vi "lib TID Path.vi"(8 "error in (no error)":errorcluster, 10 "tid":string, 11 "data path":path) -> (0 "error out":errorcluster, 1 "description":string, 2 "date":string, 3 "tid path":path, 4 "size":i64)   [LabVIEW 2014]
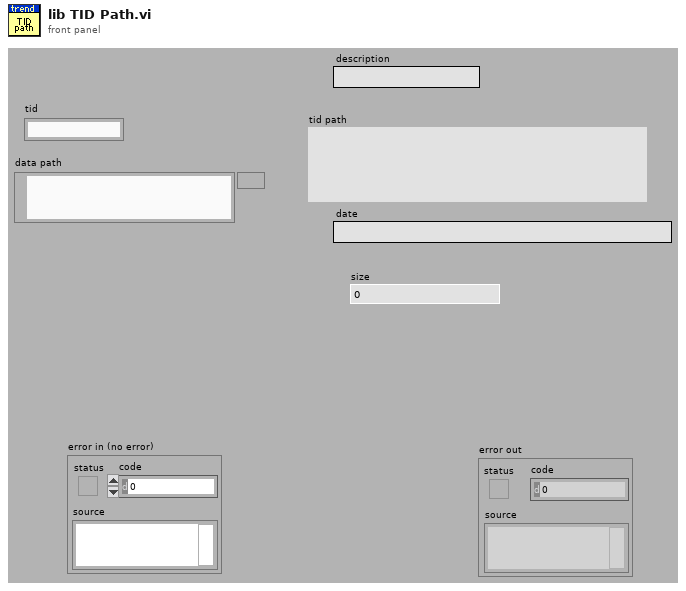
[diagram p1: front panel]
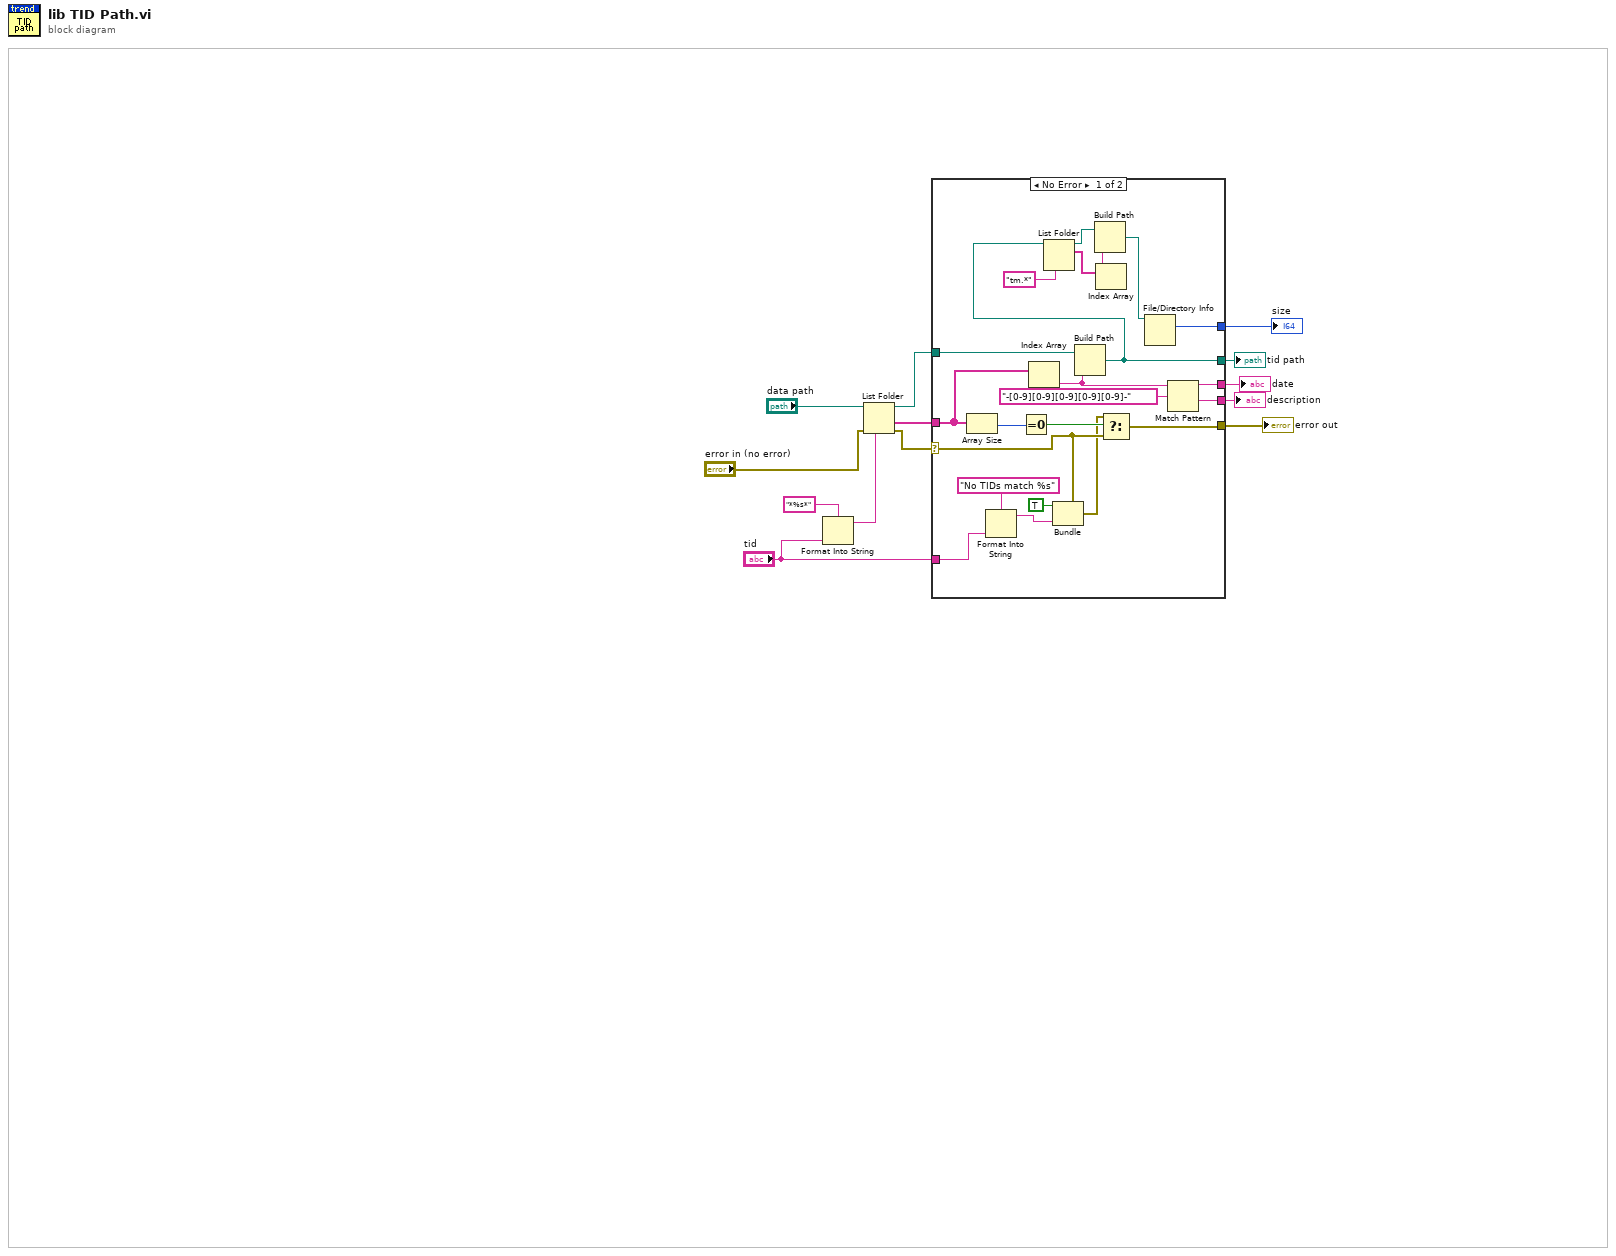
[diagram p0: block diagram]
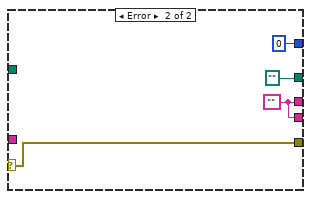
[diagram p2: hidden frame]
diagram:
  n1 = Format Into String(format string="*%s*", "tid") -> (resulting string=w10:string)  [unwired: 2 in, 1 out]
  n2 = List Folder(path="data path", pattern=w10, error in="error in (no error)") -> (path out=w7:path, folder names=w9:string[], error out=w8:errorcluster)  [unwired: 1 in, 1 out]
  n3 = case shown="No Error" w8 {
    selector: w8 -> [w28 w39]
    tunnel: w9 -> [w33 _]
    tunnel: w7 -> [w32 _]
    tunnel: [w15 path ""] -> w6
    tunnel: [w31 w39] -> w5
    tunnel: "tid" -> [w29 _]
    tunnel: [w22 w37] -> w2
    tunnel: [w21 w37] -> w3
    tunnel: [w20 i64 0 ("size")] -> w1
    frame No Error {
      n4 = Array Size(array=w33) -> (size(s)=w35:i32)
      n5 = Format Into String(format string="No TIDs match %s", w29) -> (resulting string=w27:string)  [unwired: 2 in, 1 out]
      n6 = Equal To 0?(x=w35) -> (x = 0?=w34:bool)
      n7 = Index Array(array=w33) -> (element=w24:string)  [unwired: 1 in]
      n8 = Bundle(cluster=w28, "status"=TRUE, "source"=w27) -> (w25:errorcluster)  [unwired: 1 in]
      n9 = Build Path(base path=w32, name or relative path=w24) -> (appended path=w15:path)
      n10 = List Folder(path=w15, pattern="tm.*") -> (path out=w17:path, filenames=w18:string[])  [unwired: 2 in, 2 out]
      n11 = Index Array(array=w18) -> (element=w16:string)  [unwired: 1 in]
      n12 = Build Path(base path=w17, name or relative path=w16) -> (appended path=w14:path)
      n13 = Select(t=w25, s=w34, f=w28) -> (s? t:f=w31:errorcluster)
      n14 = File/Directory Info(path=w14) -> (size=w20:i64)  [unwired: 1 in, 6 out]
      n15 = Match Pattern(string=w24, regular expression="-[0-9][0-9][0-9][0-9][0-9]-") -> (before substring=w22:string, after substring=w21:string)  [unwired: 1 in, 2 out]
    }
    frame Error {
      w37 = ""
    }
  }
  "error out" <- w5
  "tid path" <- w6
  "description" <- w3
  "date" <- w2
  "size" <- w1
